vi "FuzzyMapUnitTest.vi"() -> ()   [LabVIEW 2016]
uses:
  <vilib>/NI Modbus.llb/MB Serial Master Query Read Holding Registers (poly).vi
panel:
  out "Array 2":u16[](array[numeric])
  out "Array":i32[](array[numeric])
  out "array":string[](array[string])
  out "output array":string[](array[string])
  out "Table Control":string[][](table)
  out "Exception Code":u8 format="%.0x"
  out "error out":errorcluster
  out "Input Registers":u16[](array[numeric])
  in  "error in (no error)":errorcluster
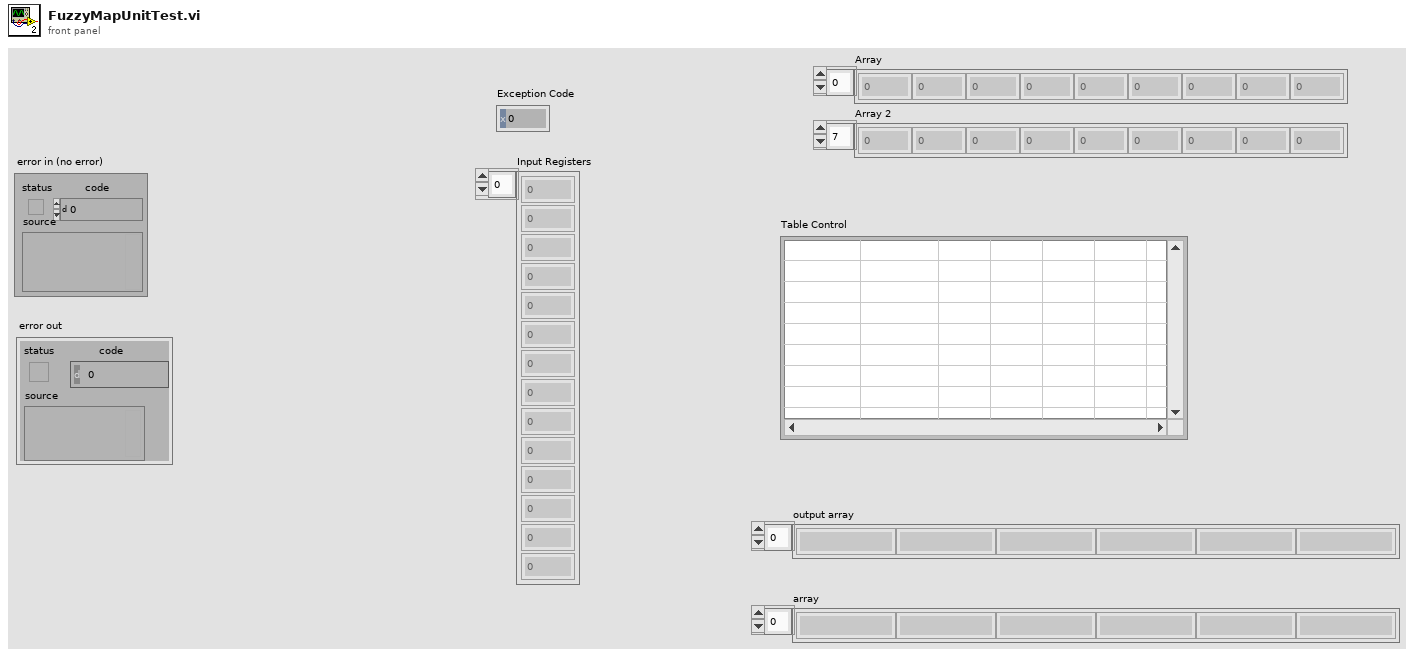
[diagram p1: front panel]
types:
  T1 = cluster{"Mode":enum16{"RTU", "ASCII"}, "Slave Address":u8}
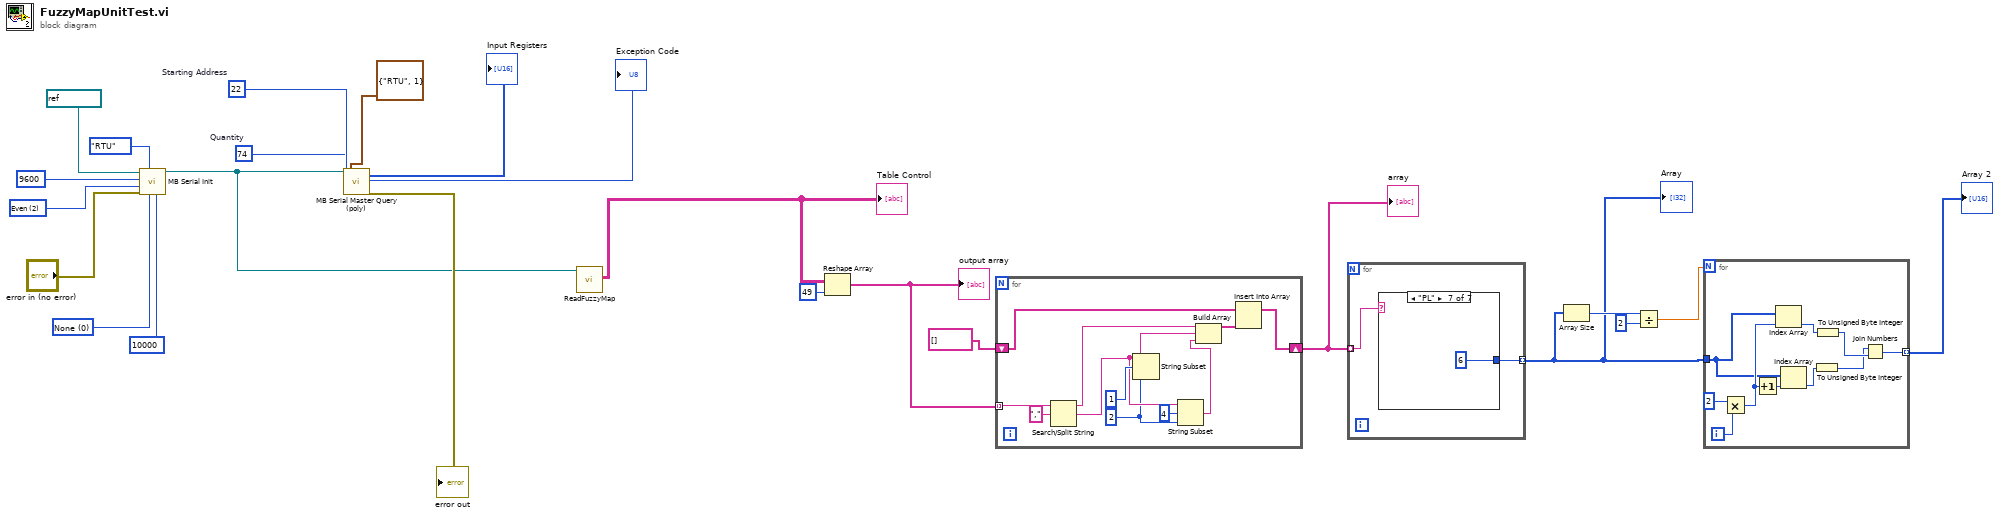
[diagram p0: block diagram]
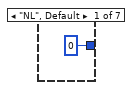
[diagram p2: hidden frame]
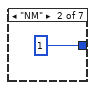
[diagram p3: hidden frame]
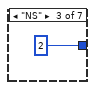
[diagram p4: hidden frame]
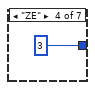
[diagram p5: hidden frame]
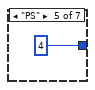
[diagram p6: hidden frame]
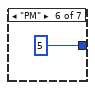
[diagram p7: hidden frame]
diagram:
  w16 = u16 74  # Quantity
  w17 = u16 22  # Starting Address
  w19 = u16 0 items=["None", "XON/XOFF", "RTS/CTS", "XON/XOFF & RTS/CTS", "DTR/DSR", "XON/XOFF & DTR/DSR"] ("Flow Control")
  w22 = u16 2 items=["None", "Odd", "Even", "Mark", "Space"] ("Parity")
  n1 = call <vilib>:"MB Serial Init.vi"("Timeout"=u32 10000, "Flow Control"=w19, "Mode"=enum16{"RTU", "ASCII"}."RTU", "error in (no error)"="error in (no error)", "Parity"=w22, "Baud Rate"=u32 9600, "VISA resource name"=refnum<visa-resource-name> "COM4") -> ("VISA resource name out"=w11:refnum<visa-resource-name>)  [unwired: 3 in, 1 out]
  n2 = call-poly <vilib>:"MB Serial Master Query (poly).vi"("VISA resource name"=w11, "Starting Address"=w17, "Quantity"=w16, "Serial Parameters"=T1 {"Mode"=enum."RTU", "Slave Address"=1}) -> ("Holding Registers"=→"Input Registers":u16[], "Exception Code"=→"Exception Code":u8, "error out"=→"error out":errorcluster)  [unwired: 12 in, 1 out]
  n3 = call "ReadFuzzyMap.vi"("VISA in"=w11) -> ("Table Control"=w10:string[][])  [unwired: 7 in, 2 out]
  "Table Control" <- w10
  n4 = Reshape Array(w10, 49 ("dimension size")) -> (w8:string[])
  "output array" <- w8
  n5 = for {
    tunnel: w8 -> [w36] mode=indexing
    shift-right: [w31] -> w6
    shift-left: string[] [] ("array") -> [w32]
    w27 = 2 ("length (rest)")
    n6 = Search/Split String(string=w36, search string/char (-)=",") -> (substring before match=w34:string, match + rest of string=w28:string)  [unwired: 1 in, 1 out]
    n7 = String Subset(string=w28, offset (0)=1, length (rest)=w27) -> (substring=w29:string)
    n8 = String Subset(string=w28, offset (0)=4, length (rest)=w27) -> (substring=w25:string)
    n9 = Build Array(w34, w29, w25) -> (w33:string[])
    n10 = Insert Into Array(array=w32, new element=w33) -> (w31:string[])  [unwired: 1 in]
  }
  "array" <- w6
  n11 = for {
    tunnel: w6 -> [w38] mode=indexing
    tunnel: [w37] -> w2 mode=indexing
    n12 = case shown="\"PL\"" w38 {
      tunnel: [0 ("length (rest)") 1 ("length (rest)") 2 ("length (rest)") 3 ("length (rest)") 4 ("length (rest)") 5 ("length (rest)") 6 ("length (rest)")] -> w37
      frame "NL", Default {
      }
      frame "NM" {
      }
      frame "NS" {
      }
      frame "ZE" {
      }
      frame "PS" {
      }
      frame "PM" {
      }
      frame "PL" {
      }
    }
  }
  "Array" <- w2
  n13 = Array Size(array=w2) -> (size(s)=w5:i32)
  n14 = Divide(x=w5, y=2) -> (x/y=w3:dbl)
  n15 = for {
    N: w3 -> [_]
    tunnel: w2 -> [w51]
    tunnel: [w48] -> w1 mode=indexing
    i -> [w55]
    n16 = Multiply(x=2, y=w55) -> (x*y=w53:i32)
    n17 = Increment(x=w53) -> (x+1=w52:i32)
    n18 = Index Array(array=w51, index=w53) -> (element=w50:i32)
    n19 = Index Array(array=w51, index=w52) -> (element=w49:i32)
    n20 = To Unsigned Byte Integer(number=w49) -> (unsigned 8bit integer=w46:u8)
    n21 = To Unsigned Byte Integer(number=w50) -> (unsigned 8bit integer=w47:u8)
    n22 = Join Numbers(hi=w46, lo=w47) -> ((hi.lo)=w48:u16)
  }
  "Array 2" <- w1
